vi "GetEquivalentKeysNumeric.vi"(8 "error in (no error)":errorcluster, 11 "KeyNumeric":i8[](array[numeric])) -> (0 "error out":errorcluster, 3 "KeysEquivalenceClassNumeric":i8[][](array[numeric]))   [LabVIEW 2020]
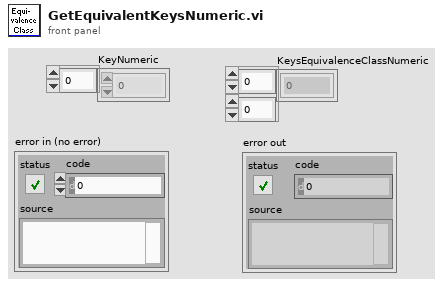
[diagram p1: front panel]
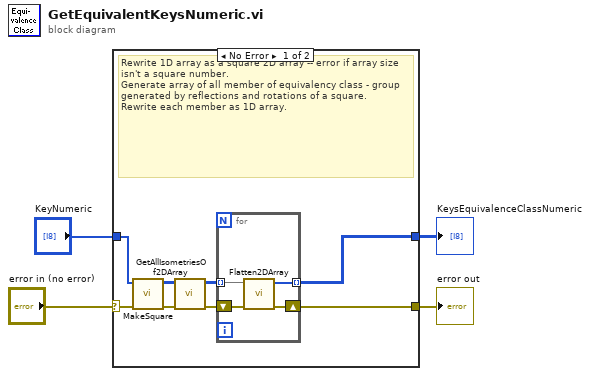
[diagram p0: block diagram]
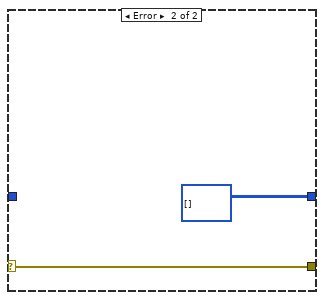
[diagram p2: hidden frame]
diagram:
  n1 = case shown="No Error" "error in (no error)" {
    selector: "error in (no error)" -> [w11 w18]
    tunnel: [w6 w18] -> w3
    tunnel: "KeyNumeric" -> [w12 _]
    tunnel: [w5 i8[][] [] ("1D Array Out")] -> w1
    frame No Error {
      # "Rewrite 1D array as a square 2D array -- error if array size isn't a square number.\nGenerate array of all member of equivalency class - group generated by reflections and rotations of a square.\nRewrite each member as 1D array."
      n2 = call "MakeSquare.vi"("error in (no error)"=w11, "KeyNumeric (Flat)"=w12) -> ("error out"=w9:errorcluster, "KeyNumeric (Square)"=w10:i8[][])  [unwired: 8 in]
      n3 = call "GetAllIsometriesOf2DArray.vi"("error in (no error)"=w9, "Array In"=w10) -> ("error out"=w7:errorcluster, "All Isometrioes Out"=w8:i8[][][])  [unwired: 8 in]
      n4 = for {
        tunnel: w8 -> [w16] mode=indexing
        shift-right: [w14] -> w6
        shift-left: w7 -> [w15]
        tunnel: [w13] -> w5 mode=indexing
        n5 = call "Flatten2DArray.vi"("error in (no error)"=w15, "2D Array In"=w16) -> ("error out"=w14:errorcluster, "1D Array Out"=w13:i8[])  [unwired: 8 in]
      }
    }
    frame Error {
    }
  }
  "KeysEquivalenceClassNumeric" <- w1
  "error out" <- w3
